vi "XLP80_CAN_MaskBytes.vi"() -> ()   [LabVIEW 2021]
panel:
  in  "DBC Settings 2":T1={"ByteOrder"=[enum."Motorola", enum."Motorola"], "Type"=[], "Factor"=[1.0, 1.0], "Offset"=[0.0, 0.0], "Startbit"=[27, 43], "Length"=[16, 16], "Mux"=[FALSE, FALSE], "Name"=["", ""]} {"Offset" format="%.3f"; "Factor" format="%.3f"}
  out "Boolean array Out 2":bool[](array[boolean])
  in  "AO Values IN 2":dbl[](array[numeric])=[65535.0, 3.0] format="%.6f"
  in  "DBC Settings":T2={"ByteOrder"=[enum."Motorola", enum."Motorola"], "Type"=[enum."Unsigned", enum."Unsigned"], "Factor"=[1.0, 1.0], "Offset"=[0.0, 0.0], "Startbit"=[27, 43], "Length"=[16, 16], "Mux"=[FALSE, FALSE]} {"Offset" format="%.3f"; "Factor" format="%.3f"}
  out "Data OUT":u8[](array[numeric])=[0, 0, 3, 32, 0, 24, 0, 0] format="%.0x"
  in  "DLC":u8=8
  out "Boolean array Out":bool[](array[boolean])=[FALSE, FALSE, FALSE, FALSE, FALSE, FALSE, FALSE, FALSE, FALSE, FALSE, FALSE, FALSE, FALSE, FALSE, FALSE, FALSE, TRUE, TRUE, FALSE, FALSE, FALSE, FALSE, FALSE, FALSE, FALSE, FALSE, FALSE, FALSE, FALSE, TRUE, FALSE, FALSE, FALSE, FALSE, FALSE, FALSE, FALSE, FALSE, FALSE, FALSE, FALSE, FALSE, FALSE, TRUE, TRUE, FALSE, FALSE, FALSE, FALSE, FALSE, FALSE, FALSE, FALSE, FALSE, FALSE, FALSE, FALSE, FALSE, FALSE, FALSE, FALSE, FALSE, FALSE, FALSE]
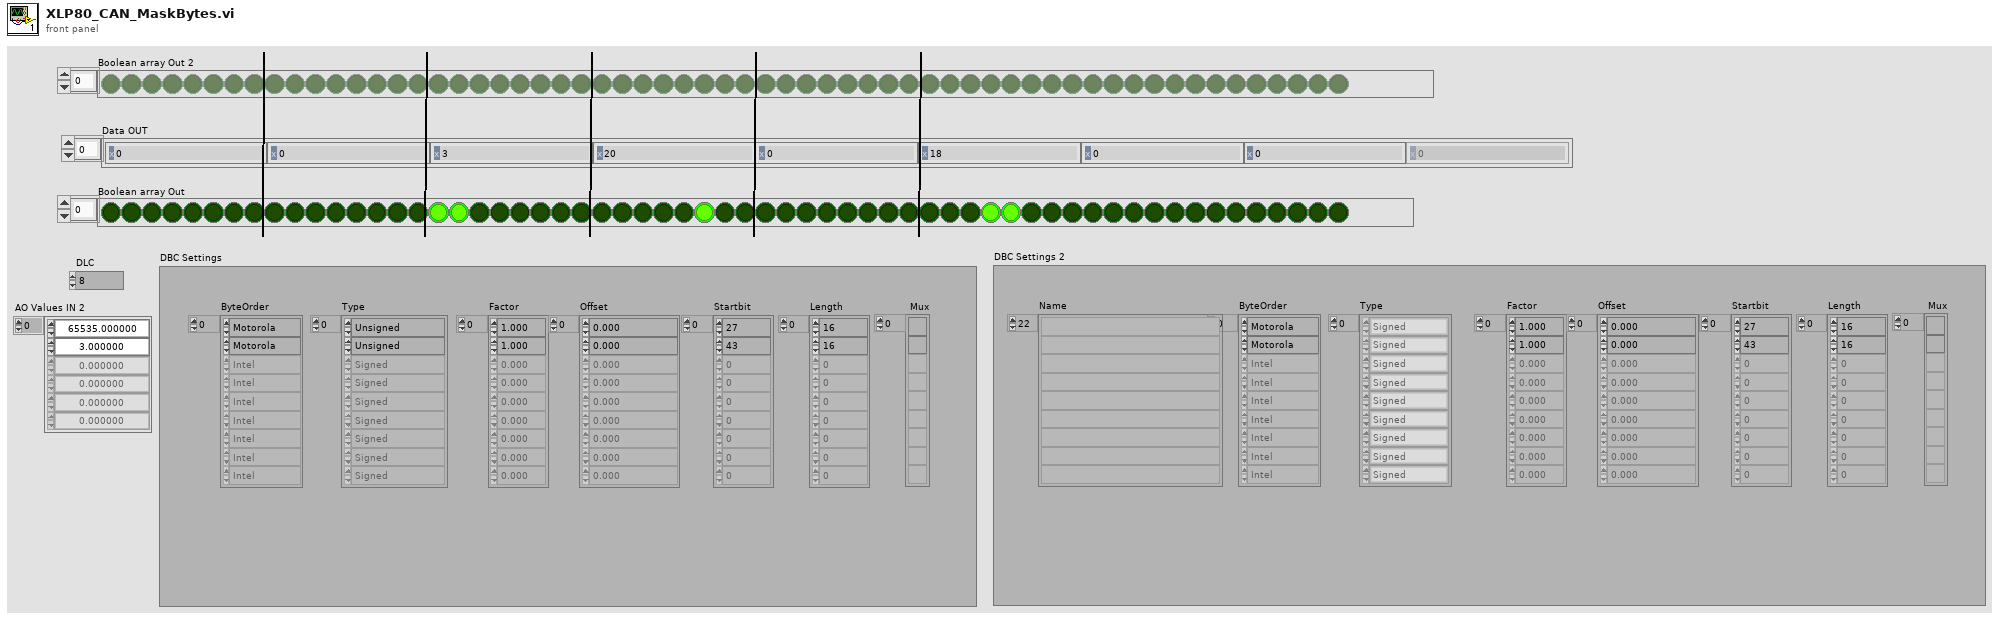
[diagram p1: front panel]
types:
  T1 = cluster{"ByteOrder":enum16{"Intel", "Motorola"}[], "Type":enum16{"Signed", "Unsigned", "IEEE Float", "Byte Array"}[], "Factor":dbl[], "Offset":dbl[], "Startbit":u32[], "Length":u32[], "Mux":bool[], "Name":string[]}
  T2 = cluster{"ByteOrder":enum16{"Intel", "Motorola"}[], "Type":enum16{"Signed", "Unsigned"}[], "Factor":dbl[], "Offset":dbl[], "Startbit":i32[], "Length":i32[], "Mux":bool[]}
  T3 = enum16{"Signed", "Unsigned", "IEEE Float", "Byte Array"}[]
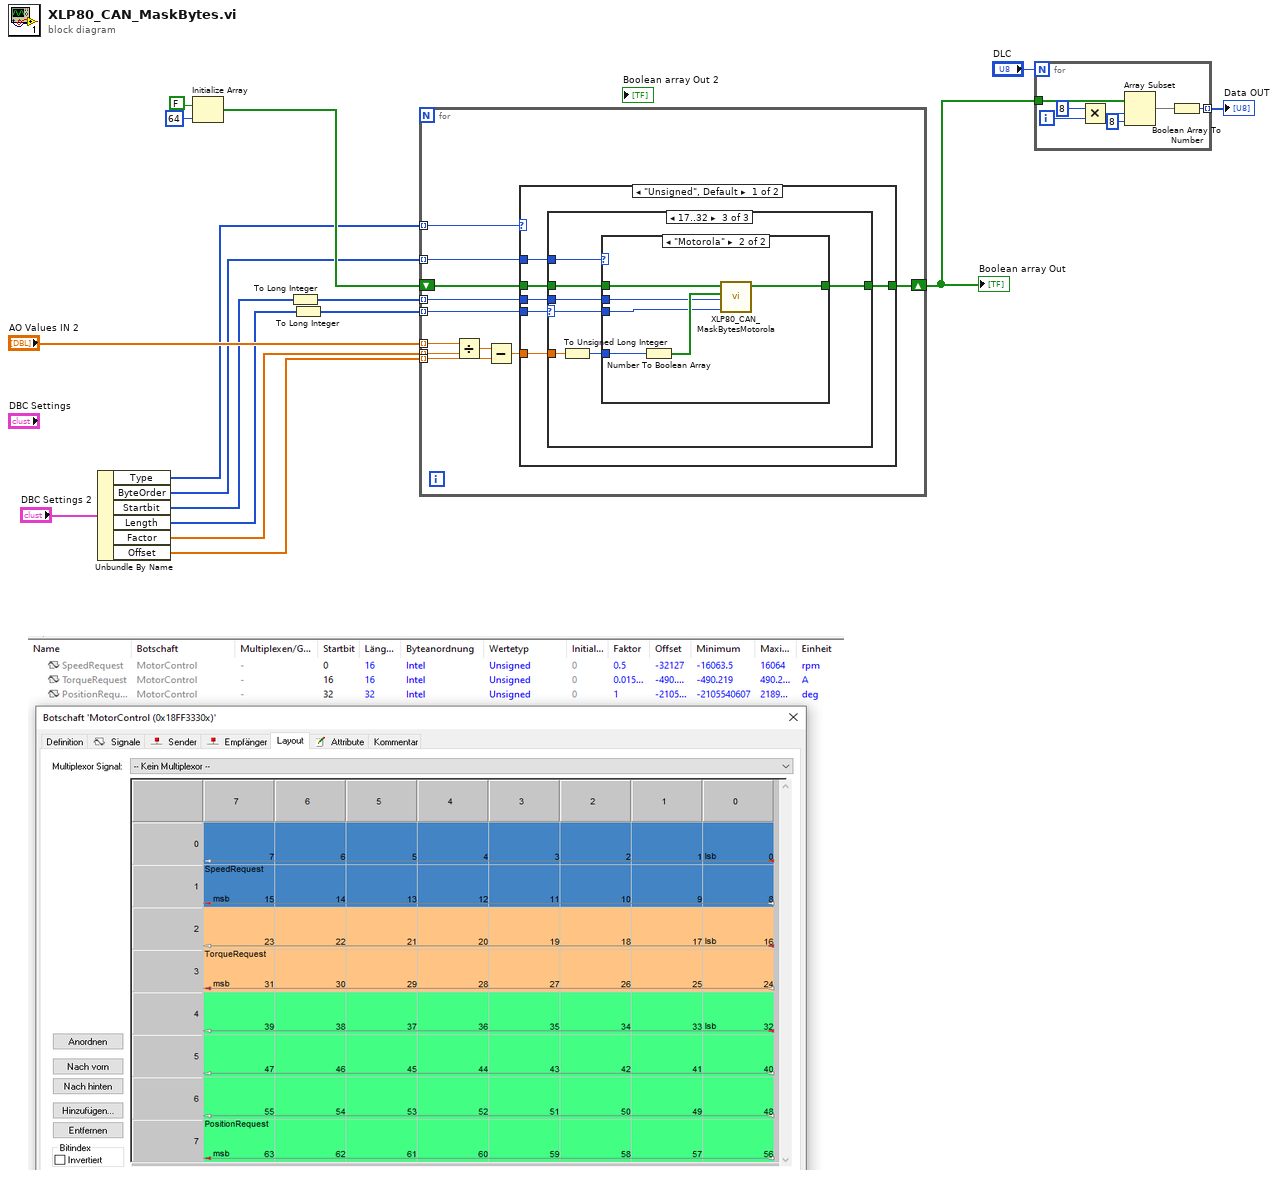
[diagram p0: block diagram]
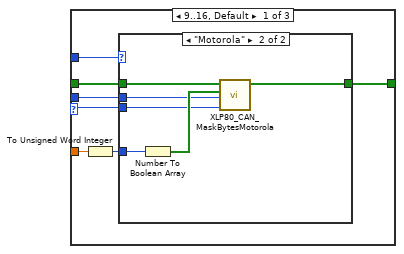
[diagram p2: hidden frame]
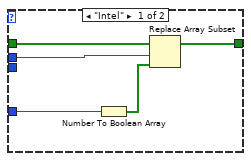
[diagram p3: hidden frame]
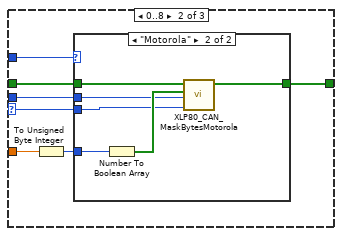
[diagram p4: hidden frame]
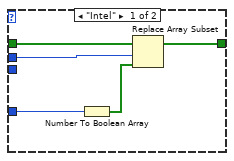
[diagram p5: hidden frame]
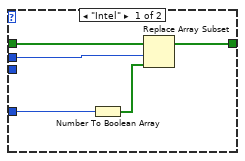
[diagram p6: hidden frame]
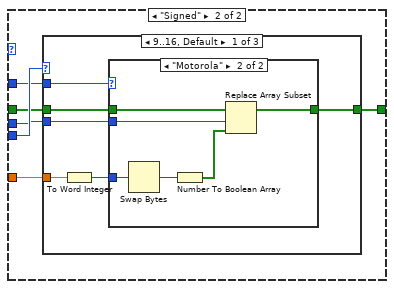
[diagram p7: hidden frame]
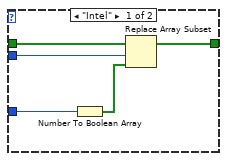
[diagram p8: hidden frame]
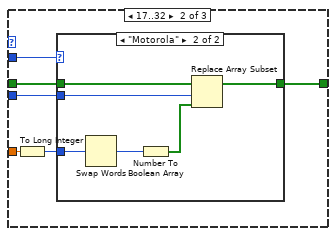
[diagram p9: hidden frame]
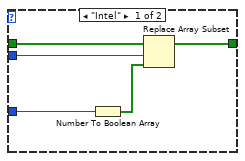
[diagram p10: hidden frame]
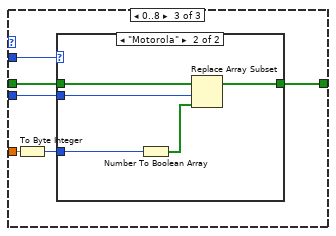
[diagram p11: hidden frame]
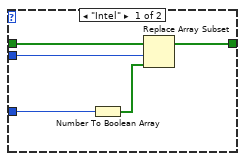
[diagram p12: hidden frame]
diagram:
  n1 = Unbundle By Name("DBC Settings 2") -> ("Type"=w7:T3, "ByteOrder"=w8:enum16{"Intel", "Motorola"}[], "Startbit"=w6:u32[], "Length"=w4:u32[], "Factor"=w2:dbl[], "Offset"=w1:dbl[])
  n2 = Initialize Array(FALSE, 64 ("dimension size")) -> (w11:bool[])
  n3 = To Long Integer(number=w6) -> (32bit integer=w5:i32[])
  n4 = To Long Integer(number=w4) -> (32bit integer=w3:i32[])
  n5 = for {
    tunnel: w2 -> [w26] mode=indexing
    tunnel: "AO Values IN 2" -> [w25] mode=indexing
    tunnel: w1 -> [w24] mode=indexing
    tunnel: w7 -> [w23] mode=indexing
    tunnel: w3 -> [w22] mode=indexing
    tunnel: w5 -> [w20] mode=indexing
    tunnel: w8 -> [w17] mode=indexing
    shift-right: [w19] -> w14
    shift-left: w11 -> [w18]
    n6 = Divide(x=w25, y=w26) -> (x/y=w27:dbl)
    n7 = Subtract(x=w27, y=w24) -> (x-y=w21:dbl)
    n8 = case shown="\"Unsigned\", Default" w23 {
      tunnel: w22 -> [w33 w93]
      tunnel: w21 -> [w32 w92]
      tunnel: w17 -> [w31 w91]
      tunnel: w18 -> [w29 w89]
      tunnel: w20 -> [w30 w90]
      tunnel: [w28 w88] -> w19
      frame "Unsigned", Default {
        n9 = case shown="17..32" w33 {
          selector: w33 -> [w34 w52 w70]
          tunnel: w32 -> [w40 w58 w76]
          tunnel: w31 -> [w39 w57 w75]
          tunnel: w30 -> [w37 w55 w73]
          tunnel: w29 -> [w36 w54 w72]
          tunnel: [w35 w53 w71] -> w28
          frame 9..16, Default {
            n10 = To Unsigned Word Integer(number=w40) -> (unsigned 16bit integer=w38:u16)
            n11 = case shown="\"Motorola\"" w39 {
              tunnel: w38 -> [w44 w49]
              tunnel: w37 -> [w41 w47]
              tunnel: w36 -> [w45 w51]
              tunnel: [w42 w50] -> w35
              tunnel: w34 -> [_ w46]
              frame "Intel" {
                n12 = Number To Boolean Array(number=w44) -> (Boolean array=w43:bool[])
                n13 = Replace Array Subset(array=w45, new element=w43, index=w41) -> (w42:bool[])
              }
              frame "Motorola" {
                n14 = Number To Boolean Array(number=w49) -> (Boolean array=w48:bool[])
                n15 = call "XLP80_CAN_MaskBytesMotorola.vi"("Length"=w46, "StartBit"=w47, "Input"=w48, "ID IN"=w51) -> ("ID OUT"=w50:bool[])  [unwired: 7 in]
              }
            }
          }
          frame 0..8 {
            n16 = To Unsigned Byte Integer(number=w58) -> (unsigned 8bit integer=w56:u8)
            n17 = case shown="\"Motorola\"" w57 {
              tunnel: w56 -> [w61 w68]
              tunnel: w55 -> [w62 w67]
              tunnel: w54 -> [w63 w66]
              tunnel: [w59 w65] -> w53
              tunnel: w52 -> [_ w64]
              frame "Intel" {
                n18 = Number To Boolean Array(number=w61) -> (Boolean array=w60:bool[])
                n19 = Replace Array Subset(array=w63, new element=w60, index=w62) -> (w59:bool[])
              }
              frame "Motorola" {
                n20 = Number To Boolean Array(number=w68) -> (Boolean array=w69:bool[])
                n21 = call "XLP80_CAN_MaskBytesMotorola.vi"("Length"=w64, "StartBit"=w67, "Input"=w69, "ID IN"=w66) -> ("ID OUT"=w65:bool[])  [unwired: 7 in]
              }
            }
          }
          frame 17..32 {
            n22 = To Unsigned Long Integer(number=w76) -> (unsigned 32bit integer=w74:u32)
            n23 = case shown="\"Motorola\"" w75 {
              tunnel: w74 -> [w79 w82]
              tunnel: w73 -> [w80 w84]
              tunnel: w72 -> [w81 w86]
              tunnel: [w77 w85] -> w71
              tunnel: w70 -> [_ w83]
              frame "Intel" {
                n24 = Number To Boolean Array(number=w79) -> (Boolean array=w78:bool[])
                n25 = Replace Array Subset(array=w81, new element=w78, index=w80) -> (w77:bool[])
              }
              frame "Motorola" {
                n26 = Number To Boolean Array(number=w82) -> (Boolean array=w87:bool[])
                n27 = call "XLP80_CAN_MaskBytesMotorola.vi"("Length"=w83, "StartBit"=w84, "Input"=w87, "ID IN"=w86) -> ("ID OUT"=w85:bool[])  [unwired: 7 in]
              }
            }
          }
        }
      }
      frame "Signed" {
        n28 = case shown="9..16, Default" w93 {
          tunnel: w92 -> [w99 w116 w133]
          tunnel: w91 -> [w98 w115 w132]
          tunnel: w90 -> [w96 w113 w130]
          tunnel: w89 -> [w95 w112 w129]
          tunnel: [w94 w111 w128] -> w88
          frame 9..16, Default {
            n29 = To Word Integer(number=w99) -> (16bit integer=w97:i16)
            n30 = case shown="\"Motorola\"" w98 {
              tunnel: w97 -> [w102 w108]
              tunnel: w96 -> [w103 w109]
              tunnel: w95 -> [w104 w110]
              tunnel: [w100 w106] -> w94
              frame "Intel" {
                n31 = Number To Boolean Array(number=w102) -> (Boolean array=w101:bool[])
                n32 = Replace Array Subset(array=w104, new element=w101, index=w103) -> (w100:bool[])
              }
              frame "Motorola" {
                n33 = Swap Bytes(anything=w108) -> (byte swapped=w105:i16)
                n34 = Number To Boolean Array(number=w105) -> (Boolean array=w107:bool[])
                n35 = Replace Array Subset(array=w110, new element=w107, index=w109) -> (w106:bool[])
              }
            }
          }
          frame 17..32 {
            n36 = To Long Integer(number=w116) -> (32bit integer=w114:i32)
            n37 = case shown="\"Motorola\"" w115 {
              tunnel: w114 -> [w119 w125]
              tunnel: w113 -> [w120 w126]
              tunnel: w112 -> [w121 w127]
              tunnel: [w117 w123] -> w111
              frame "Intel" {
                n38 = Number To Boolean Array(number=w119) -> (Boolean array=w118:bool[])
                n39 = Replace Array Subset(array=w121, new element=w118, index=w120) -> (w117:bool[])
              }
              frame "Motorola" {
                n40 = Swap Words(1:w125) -> (0:w122:i32)
                n41 = Number To Boolean Array(number=w122) -> (Boolean array=w124:bool[])
                n42 = Replace Array Subset(array=w127, new element=w124, index=w126) -> (w123:bool[])
              }
            }
          }
          frame 0..8 {
            n43 = To Byte Integer(number=w133) -> (8bit integer=w131:i8)
            n44 = case shown="\"Motorola\"" w132 {
              tunnel: w131 -> [w136 w139]
              tunnel: w130 -> [w137 w142]
              tunnel: w129 -> [w138 w143]
              tunnel: [w134 w140] -> w128
              frame "Intel" {
                n45 = Number To Boolean Array(number=w136) -> (Boolean array=w135:bool[])
                n46 = Replace Array Subset(array=w138, new element=w135, index=w137) -> (w134:bool[])
              }
              frame "Motorola" {
                n47 = Number To Boolean Array(number=w139) -> (Boolean array=w141:bool[])
                n48 = Replace Array Subset(array=w143, new element=w141, index=w142) -> (w140:bool[])
              }
            }
          }
        }
      }
    }
  }
  "Boolean array Out" <- w14
  n49 = for {
    N: "DLC" -> [_]
    tunnel: w14 -> [w150]
    tunnel: [w144] -> w15 mode=indexing
    i -> [w149]
    n50 = Multiply(x=8, y=w149) -> (x*y=w148:i32)
    n51 = Array Subset(array=w150, index=w148, length=8) -> (w145:bool[])
    n52 = Boolean Array To Number(Boolean array=w145) -> (number=w144:u8)
  }
  "Data OUT" <- w15
